vi "Add authenticator.vi"(7 "Authentication Method":T1, 8 "error in (no error)":errorcluster, 9 "Secret":string, 10 "Authentication ID":string, 11 "WAMP Client in":refnum<class "WAMP Client.lvclass">) -> (0 "error out":errorcluster, 3 "WAMP Client out":refnum<class "WAMP Client.lvclass">)   [LabVIEW 2020, in "wamplv.lvlib" / "WAMP Client.lvclass"]
uses:
  WAMP Client.lvclass
  TypeDef/Authentication Method.ctl
  WAMP Client.lvclass/WAMP Client.ctl
  Private/Authenticators/TicketAuthentactor/TicketAuthentactor.lvclass
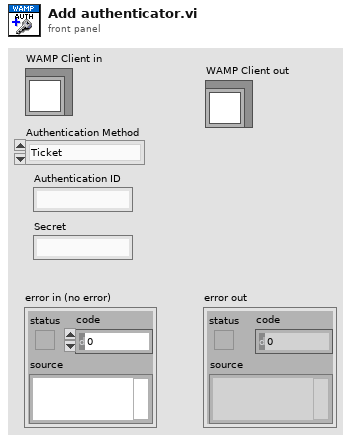
[diagram p1: front panel]
types:
  T1 = typedef "wamplv.lvlib/WAMP Client.lvclass/Authentication Method.ctl" = enum16{"Ticket"}
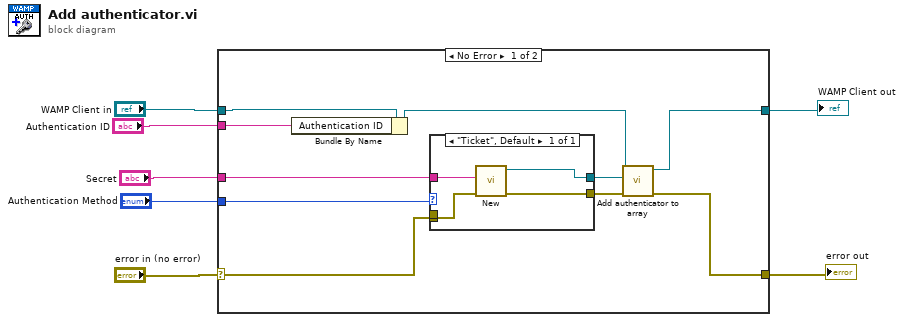
[diagram p0: block diagram]
diagram:
  n1 = case shown="No Error" "error in (no error)" {
    selector: "error in (no error)" -> [w17 w23]
    tunnel: [w13 w23] -> w6
    tunnel: [w15 w22] -> w4
    tunnel: "WAMP Client in" -> [w10 w22]
    tunnel: "Authentication Method" -> [w12 _]
    tunnel: "Secret" -> [w11 _]
    tunnel: "Authentication ID" -> [w8 _]
    frame No Error {
      n2 = Bundle By Name(cluster=w10, "Authentication ID"=w8) -> (w9:refnum<class "WAMP Client.lvclass">)
      n3 = case shown="\"Ticket\", Default" w12 {
        tunnel: w17 -> [w18]
        tunnel: [w21] -> w16
        tunnel: [w20] -> w14
        tunnel: w11 -> [w19]
        tunnel: [w18] -> _
        frame "Ticket", Default {
          n4 = call "New.vi"("error in (no error)"=w18, "Secret"=w19) -> ("error out"=w20:errorcluster, "TicketAuthentactor out"=w21:refnum<class "TicketAuthentactor.lvclass">)  [unwired: 8 in]
        }
      }
      n5 = call "Add authenticator to array.vi"("error in (no error)"=w14, "TicketAuthentactor in"=w16, "WAMP Client in"=w9) -> ("error out"=w13:errorcluster, "WAMP Client out"=w15:refnum<class "WAMP Client.lvclass">)  [unwired: 7 in]
    }
    frame Error {
    }
  }
  "error out" <- w6
  "WAMP Client out" <- w4
